vi "Benchtop Piezo Example.vi"() -> ()   [LabVIEW 2012]
uses:
  U:/Kinesis LabVIEW Alpha/Thorlabs.MotionControl.Controls.dll
  Thorlabs.MotionControl.Controls.dll
  U:/Kinesis LabVIEW Alpha/Thorlabs.MotionControl.Benchtop.PiezoCLI.dll
  Thorlabs.MotionControl.Benchtop.PiezoCLI.dll
  U:/Kinesis LabVIEW Alpha/Thorlabs.MotionControl.GenericPiezoCLI.dll
  Thorlabs.MotionControl.GenericPiezoCLI.dll
panel:
  out "GetOutputVoltage":dbl
  in  "stop":bool
  in  "BenchtopPiezoControl":refnum<k24>(container)
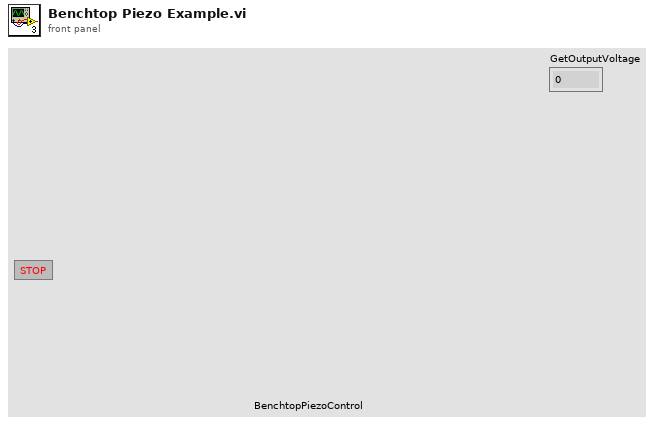
[diagram p1: front panel]
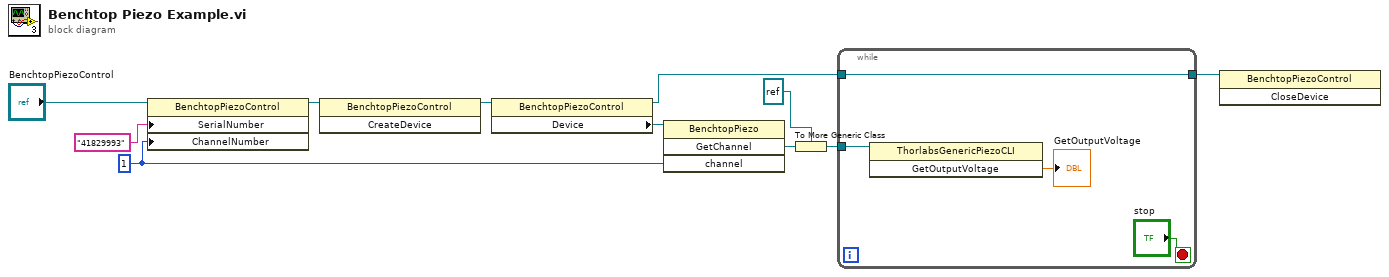
[diagram p0: block diagram]
diagram:
  w5 = 1 ("ChannelNumber")
  n1 = property class="BenchtopPiezoControl"(reference="BenchtopPiezoControl", "SerialNumber"="41829993", "ChannelNumber"=w5) -> (reference out=w9:refnum<k24>)  [unwired: 1 in, 1 out]
  n2 = invoke class="BenchtopPiezoControl" method="CreateDevice"(reference=w9) -> (reference out=w8:refnum<k24>)  [unwired: 2 in, 2 out]
  n3 = property class="BenchtopPiezoControl"(reference=w8) -> (reference out=w6:refnum<k24>, "Device"=w3:refnum<k24>)  [unwired: 1 in, 1 out]
  n4 = invoke class="BenchtopPiezo" method="GetChannel"(reference=w3, "channel"=w5) -> ("GetChannel"=w4:refnum<k24>)  [unwired: 2 in, 3 out]
  n5 = To More Generic Class(target class=refnum<k24> refnum, reference=w4) -> (generic class reference=w1:refnum<k24>)
  n6 = while {
    tunnel: [w14] -> w7
    tunnel: w6 -> [w14]
    tunnel: w1 -> [w13]
    stop <- "stop" stop-if-true
    n7 = invoke class="ThorlabsGenericPiezoCLI" method="GetOutputVoltage"(reference=w13) -> ("GetOutputVoltage"=→"GetOutputVoltage":dbl)  [unwired: 2 in, 2 out]
  }
  n8 = invoke class="BenchtopPiezoControl" method="CloseDevice"(reference=w7) -> ()  [unwired: 2 in, 3 out]
